vi "Get Name.vi"(11 "CD Template":refnum<class "NIVS_Asynchronous Timing and Sync.lvclass">) -> (2 "String":string)   [LabVIEW 2019, in "NIVS_Asynchronous Timing and Sync.lvclass"]
uses:
  NIVS_Asynchronous Timing and Sync.lvclass
  NIVS_Consolidated_CDW_MetaDataObj/Execution Mode.ctl
  NIVS_Consolidated_CDW_MetaDataObj/NIVS_Consolidated_CDW_MetaDataObj.lvclass
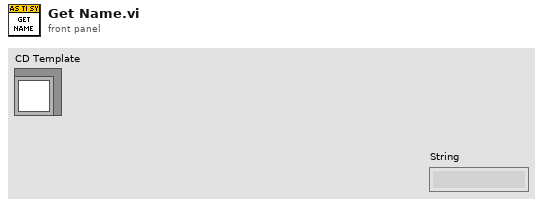
[diagram p1: front panel]
types:
  T1 = typedef "NIVS_Consolidated_CDW_MetaDataObj.lvclass/Execution Mode.ctl" = enum16{"Asynchronous", "Inline HW Interface", "Inline Model Interface", "Inline Timing and Sync", "Asynchronous Timing and Sync"}
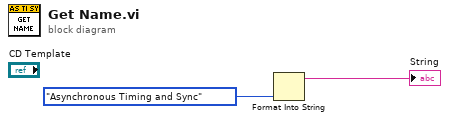
[diagram p0: block diagram]
diagram:
  n1 = Format Into String(Execution_Mode."Asynchronous Timing and Sync" ("CD Execution Mode")) -> (resulting string=→"String":string)  [unwired: 3 in, 1 out]
